vi "Voltage - White Noise - Corrected - NI.vi"() -> ()   [LabVIEW 2022 SP3]
doc: "This example demonstrates how to continuously re-generate analog output data from a buffer in your computer's memory.\n\nRefer to your device documentation for pinouts and hardware capabilities."
uses:
  WhiteNoise.ctl
  <vilib>/Utility/error.llb/DialogType.ctl
  <vilib>/DAQmx/write.llb/DAQmx Write (Analog 1D Wfm NChan NSamp).vi
  <vilib>/DAQmx/create/channels.llb/DAQmx Create Channel (AO-Voltage-Basic).vi
  <vilib>/DAQmx/configure/timing.llb/DAQmx Timing (Sample Clock).vi
  <vilib>/measure/maspectr.llb/FFT Spectrum (Mag-Phase) for N Chan.vi
  <vilib>/DAQmx/miscellaneous.llb/DAQmx Fill In Error Info.vi
  <resource>/objmgr/daqmx.rc
  <vilib>/measure/NI_MABase.lvlib
  <vilib>/measure/NI_MAPro.lvlib
panel:
  in  "?":enum32{"White Noise", "Harmonic"}(tab)
  in  "Cluster":T2={"Seed"=0.0, "Standard Deviation"=1.0, "Reset"=FALSE, "Iterator"=1.0} {"Standard Deviation" format="%0.2p"}
  in  "Cluster 2":T3={"Iterator"=1.0, "Waveform Type"=0, "Frequency"=10.0, "Amplitude"=0.5} {"Amplitude" format="%0.2p"; "Frequency" format="%0.2p"; "Waveform Type" items=["Sine Wave", "Triangle Wave", "Square Wave", "Sawtooth Wave"]}
  in  "Reset Averaging":bool
  out "Phase":cluster{"f0":dbl, "df":dbl, "phase":dbl[]}[](graph)
  out "Mag":cluster{"f0":dbl, "df":dbl, "magnitude":dbl[]}[](graph)
  in  "Number of Samples":i32=40000
  in  "Stop":bool
  out "Waveform Graph":waveform(dbl)[](graph)=[{"t0"=timestamp(0 s since 1904-01-01), "dt"=0.001, "Y"=[]}]
  in  "Sample Rate":dbl=41200.0
  in  "Sample Clock Source":tag="OnboardClock"
  in  "Max Voltage":dbl=3.5
  in  "Min Voltage":dbl=-3.5
  in  "Physical Channel(s)":tag="NI-USB-4431/ao0"
  out "Actual Sample Rate":dbl=1000.0 format="%0.2f"
  # "Channel Settings"
  # "Output"
  # "Timing and\nBuffer Settings"
  # "Waveform Settings"
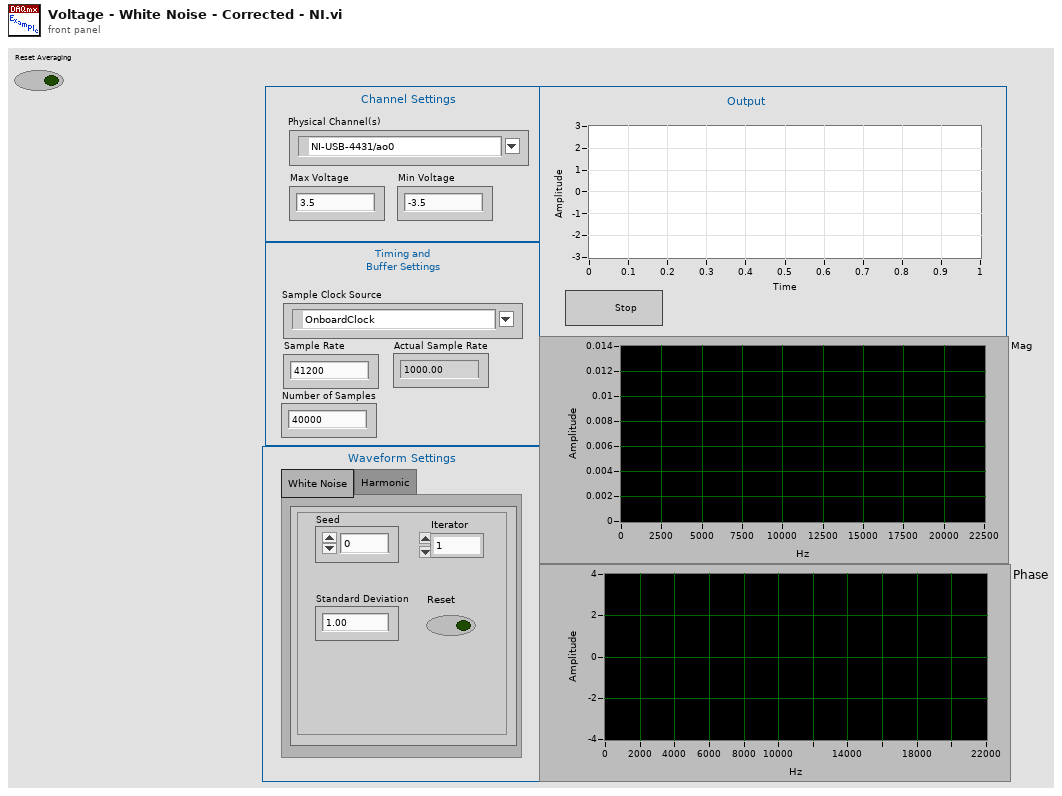
[diagram p1: front panel]
types:
  T1 = typedef "WhiteNoise.ctl" = dbl
  T2 = cluster{"Seed":T1, "Standard Deviation":dbl, "Reset":bool, "Iterator":dbl}
  T3 = cluster{"Iterator":dbl, "Waveform Type":u16, "Frequency":dbl, "Amplitude":dbl}
  T4 = typedef "DialogType.ctl" = u16
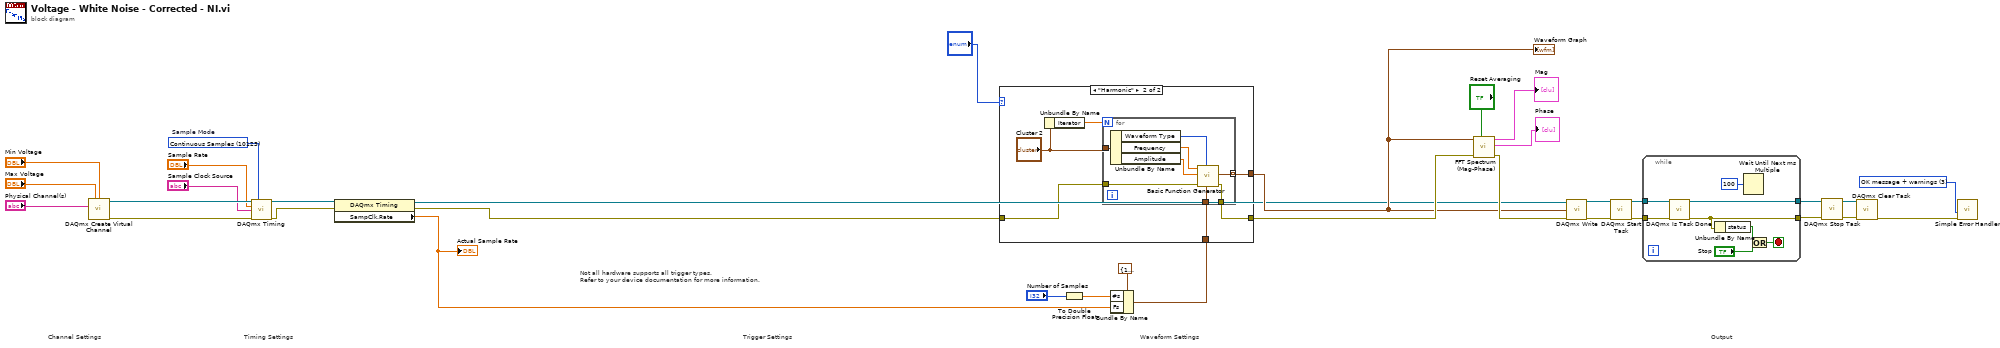
[diagram p0: block diagram]
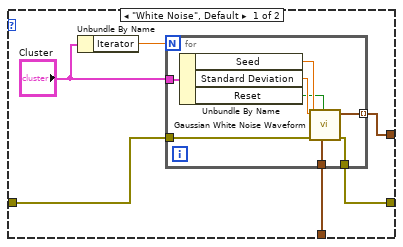
[diagram p2: hidden frame]
diagram:
  w11 = T4 3 items=["no dialog", "OK message", "continue or stop message", "OK message + warnings", "continue/stop + warnings"] ("type of dialog (OK msg:1)")
  w32 = 10123 items=["Finite Samples"=10178, "Continuous Samples"=10123, "Hardware Timed Single Point"=12522]  # Sample Mode
  # "Trigger Settings"
  # "Not all hardware supports all trigger types.\nRefer to your device documentation for more information."
  # "Output"
  # "Waveform Settings"
  # "Timing Settings"
  # "Channel Settings"
  n1 = call-poly <vilib>:"DAQmx Create Virtual Channel.vi"("maximum value"="Max Voltage", "minimum value"="Min Voltage", "physical channels"="Physical Channel(s)") -> ("task out"=w30:refnum<k21>, "error out"=w31:errorcluster)  [unwired: 11 in]
  n2 = call-poly <vilib>:"DAQmx Timing.vi"("task/channels in"=w30, "sample mode"=w32, "rate"="Sample Rate", "source"="Sample Clock Source", "error in"=w31) -> ("task out"=w34:refnum<k21>, "error out"=w33:errorcluster)  [unwired: 9 in]
  n3 = property class="DAQmx Timing"(reference=w34, error in=w33) -> (reference out=w2:refnum<k21>, error out=w1:errorcluster, "SampClk.Rate"=w20:dbl)
  "Actual Sample Rate" <- w20
  n4 = To Double Precision Float(number="Number of Samples") -> (double precision float=w17:dbl)
  n5 = Bundle By Name(cluster=cluster{"Fs":dbl, "#s":dbl} {"Fs"=1000.0, "#s"=1000.0} ("sampling info"), "#s"=w17, "Fs"=w20) -> (w19:cluster{"Fs":dbl, "#s":dbl})
  n6 = case shown="\"Harmonic\"" "?" {
    tunnel: w19 -> [w40 w52]
    tunnel: w1 -> [w39 w54]
    tunnel: [w38 w51] -> w5
    tunnel: [w35 w53] -> w4
    frame "White Noise", Default {
      n7 = Unbundle By Name("Cluster") -> ("Iterator"=w37:dbl)
      n8 = for {
        N: w37 -> [_]
        tunnel: w39 -> [w48]
        tunnel: w40 -> [w47]
        tunnel: [w46] -> w38
        tunnel: "Cluster" -> [w45]
        tunnel: [w44] -> w35 mode=indexing
        n9 = Unbundle By Name(w45) -> ("Seed"=w43:T1, "Standard Deviation"=w42:dbl, "Reset"=w41:bool)
        n10 = call <vilib>:"Gaussian White Noise Waveform.vi"("sampling info"=w47, "reset signal"=w41, "error in (no error)"=w48, "seed"=w43, "standard deviation"=w42) -> ("error out"=w46:errorcluster, "signal out"=w44:waveform(dbl))  [unwired: 5 in]
      }
    }
    frame "Harmonic" {
      n11 = Unbundle By Name("Cluster 2") -> ("Iterator"=w50:dbl)
      n12 = for {
        N: w50 -> [_]
        tunnel: w54 -> [w62]
        tunnel: w52 -> [w61]
        tunnel: [w60] -> w51
        tunnel: "Cluster 2" -> [w59]
        tunnel: [w55] -> w53 mode=indexing
        n13 = Unbundle By Name(w59) -> ("Waveform Type"=w58:u16, "Frequency"=w57:dbl, "Amplitude"=w56:dbl)
        n14 = call <vilib>:"Basic Function Generator.vi"("sampling info"=w61, "signal type"=w58, "error in (no error)"=w62, "amplitude"=w56, "frequency"=w57) -> ("error out"=w60:errorcluster, "signal out"=w55:waveform(dbl))  [unwired: 4 in, 1 out]
      }
    }
  }
  "Waveform Graph" <- w4
  n15 = call-poly <vilib>:"FFT Spectrum (Mag-Phase).vi"("restart averaging (F)"="Reset Averaging", "error in (no error)"=w5, "time signals"=w4) -> ("error out"=w6:errorcluster, "phases"=→"Phase":cluster{"f0":dbl, "df":dbl, "phase":dbl[]}[], "magnitudes"=→"Mag":cluster{"f0":dbl, "df":dbl, "magnitude":dbl[]}[])  [unwired: 4 in, 2 out]
  n16 = call-poly <vilib>:"DAQmx Write.vi"("task/channels in"=w2, "data"=w4, "error in"=w6) -> ("task out"=w18:refnum<k21>, "error out"=w10:errorcluster)  [unwired: 10 in, 1 out]
  n17 = call <vilib>:"DAQmx Start Task.vi"("task/channels in"=w18, "error in"=w10) -> ("task out"=w29:refnum<k21>, "error out"=w28:errorcluster)  [unwired: 12 in]
  n18 = while {
    tunnel: w29 -> [w70]
    tunnel: w28 -> [w69]
    tunnel: [w66] -> w12
    tunnel: [w67] -> w13
    stop <- w68 stop-if-true
    n19 = call <vilib>:"DAQmx Is Task Done.vi"("task/channels in"=w70, "error in"=w69) -> ("task out"=w67:refnum<k21>, "error out"=w66:errorcluster)  [unwired: 11 in, 1 out]
    n20 = Unbundle By Name(w66) -> ("status"=w65:bool)
    n21 = Wait Until Next ms Multiple(millisecond multiple=u32 100) -> ()  [unwired: 1 out]
    n22 = Or(x=w65, y="Stop") -> (x .or. y?=w68:bool)
  }
  n23 = call <vilib>:"DAQmx Stop Task.vi"("task/channels in"=w13, "error in"=w12) -> ("task out"=w15:refnum<k21>, "error out"=w14:errorcluster)  [unwired: 12 in]
  n24 = call <vilib>:"DAQmx Clear Task.vi"("task in"=w15, "error in"=w14) -> ("error out"=w27:errorcluster)  [unwired: 13 in]
  n25 = call <vilib>:"Simple Error Handler.vi"("type of dialog (OK msg:1)"=w11, "error in (no error)"=w27) -> ()  [unwired: 3 in, 5 out]
